vi "Replace SubVI (by Name).vi"(7 "SubVI to replace with":string, 8 "error in (no error)":errorcluster, 9 "SubVI being replaced":string, 10 "VI in":refnum<vi>, 11 "Library in":refnum<vi>) -> (0 "error out":errorcluster, 2 "VI out":refnum<vi>, 3 "Library out":refnum<vi>)   [LabVIEW 2019, in "gRPC Template Creation Utility.lvlib"]
uses:
  gRPC Template Creation Utility.lvlib
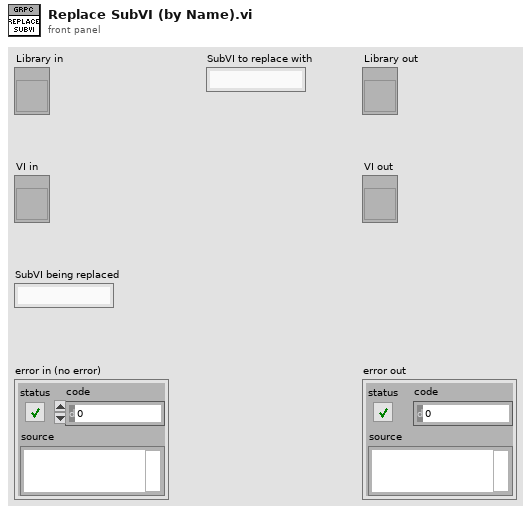
[diagram p1: front panel]
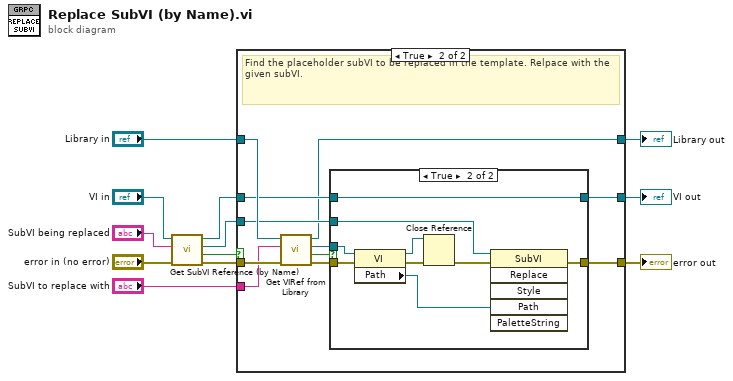
[diagram p0: block diagram]
diagram:
  n1 = call "Get SubVI Reference (by Name).vi"("error in (no error)"="error in (no error)", "SubVI Name"="SubVI being replaced", "Owner VI in"="VI in") -> ("error out"=w8:errorcluster, "Found ?"=w4:bool, "SubVI Refnum out"=w5:refnum<vi>, "Owner VI out"=w7:refnum<vi>)  [unwired: 5 in]
  n2 = case shown="True" w4 {
    tunnel: w5 -> [_ w22]
    tunnel: "Library in" -> [w13 w26]
    tunnel: w7 -> [w15 w23]
    tunnel: [w15 w21] -> w9
    tunnel: w8 -> [w14 w20]
    tunnel: [w14 w18] -> w11
    tunnel: [w13 w17] -> w10
    tunnel: "SubVI to replace with" -> [_ w16]
    frame False {
    }
    frame True {
      # "Find the placeholder subVI to be replaced in the template. Relpace with the given subVI."
      n3 = call "Get VIRef from Library.vi"("error in (no error)"=w20, "item name"=w16, "library in"=w26) -> ("error out"=w19:errorcluster, "found"=w25:bool, "vi"=w24:refnum<vi>, "library out"=w17:refnum<vi>)  [unwired: 5 in]
      n4 = case shown="True" w25 {
        tunnel: w24 -> [_ w37]
        tunnel: w23 -> [w28 w33]
        tunnel: w22 -> [_ w36]
        tunnel: [w28 w33] -> w21
        tunnel: w19 -> [w27 w32]
        tunnel: [w27 w34] -> w18
        frame False {
        }
        frame True {
          n5 = property class="VI"(reference=w37, error in=w32) -> (reference out=w30:refnum<vi>, error out=w31:errorcluster, "Path"=w35:path)
          n6 = Close Reference(reference=w30, error in (no error)=w31) -> (error out=w29:errorcluster)
          n7 = invoke class="SubVI" method="Replace"(reference=w36, error in=w29, "Path"=w35) -> (error out=w34:errorcluster)  [unwired: 3 in, 5 out]
        }
      }
    }
  }
  "error out" <- w11
  "Library out" <- w10
  "VI out" <- w9
